vi "CLD 8 CSV file commands utility Exercise.vi"(8 "Error In":errorcluster) -> (0 "Error Out":errorcluster, 3 "Commands Out Array":T1[](array[typedef]))   [LabVIEW 2015]
doc: "CLD 8 exercise"
uses:
  <vilib>/Utility/file.llb/Read Delimited Spreadsheet (string).vi
  CLD 8 Data Cluster.ctl
panel:
  in  "stop":bool
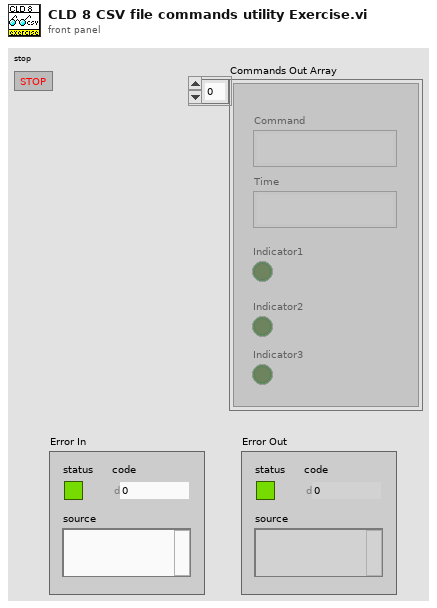
[diagram p1: front panel]
types:
  T1 = typedef "CLD 8 Data Cluster.ctl" = cluster{"Command":string, "Time":string, "Indicator1":bool, "Indicator2":bool, "Indicator3":bool}
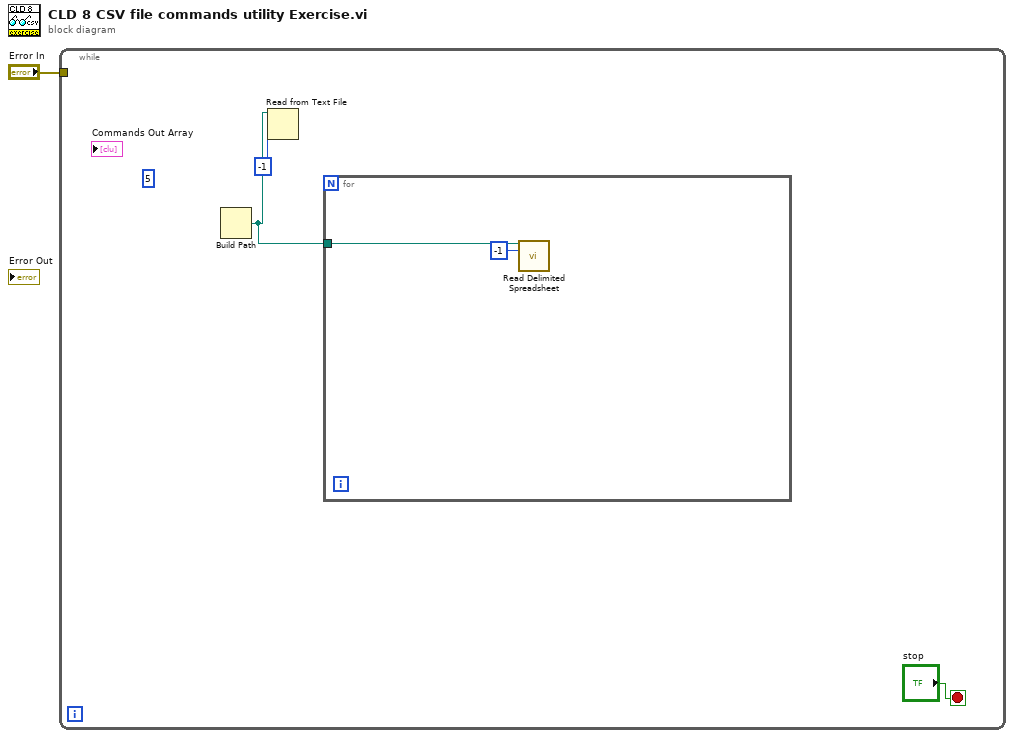
[diagram p0: block diagram]
diagram:
  n1 = while {
    tunnel: "Error In" -> [_]
    stop <- "stop" stop-if-true
    (unwired) 5 ("number of rows (all:-1)")
    n2 = Build Path() -> (appended path=w3:path)  [unwired: 2 in]
    n3 = Read from Text File(file (use dialog)=w3, count=-1) -> ()  [unwired: 2 in, 4 out]
    n4 = for {
      tunnel: w3 -> [w6]
      n5 = call-poly <vilib>:"Read Delimited Spreadsheet.vi"("file path (dialog if empty)"=w6, "number of rows (all:-1)"=-1) -> ()  [unwired: 8 in, 6 out]
    }
  }
